vi "ELVIS III v1.0 Build Bitmask DIO.vi"(10 "bool Value List In":bool[](array[boolean]), 11 "Channel List":T3) -> (1 "Bitmask to Channel Array":T1[](array[typedef]), 2 "OUT Bitmask Array":bool[][](array[boolean]), 3 "DIR Bitmask Array":bool[][](array[boolean]))   [LabVIEW 2021]
uses:
  <vilib>/myRIO/Common/Instrument Driver Framework/myRIO v1.0/DIO/typedefs/DIO Channels List.ctl
  <vilib>/myRIO/Common/Instrument Driver Framework/myRIO v1.0/DIO/typedefs/DIO Channels Enum.ctl
  <vilib>/myRIO/Common/Instrument Driver Framework/ELVIS III v1.0/DIO/typedefs/ELVIS III DIO Bitmask to Channel Map.ctl
  <vilib>/myRIO/Common/Instrument Driver Framework/ELVIS III v1.0/DIO/typedefs/ELVIS III DIO Bank Enum.ctl
panel:
  # "This VI is used by both the myRIO v1.0 Read DIO and Write DIO VIs. \nIf a bool Value List in is provided the appropriate OUT Botmask Array will be generated, otherwise all values in the array will be false."
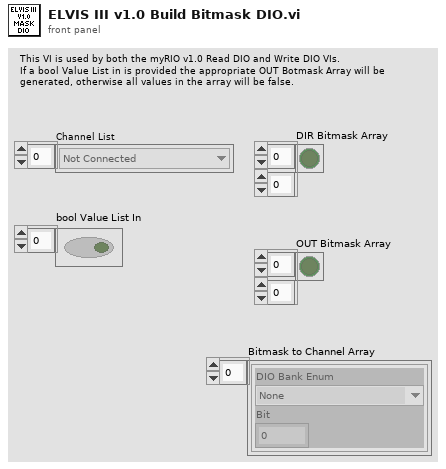
[diagram p1: front panel]
types:
  T1 = typedef "ELVIS III DIO Bitmask to Channel Map.ctl" = cluster{"DIO Bank Enum":T2, "Bit":i32}
  T2 = typedef "ELVIS III DIO Bank Enum.ctl" = enum32{"None", "A/DIO19:0", "B/DIO19:0", "LED3:0", "Button0"}
  T3 = typedef "DIO Channels List.ctl" = T4[]
  T4 = typedef "DIO Channels Enum.ctl" = enum16{"Not Connected", "C/DIO0", "C/DIO1", "C/DIO2", "C/DIO3", "C/DIO4", "C/DIO5", "C/DIO6", "C/DIO7", "A/DIO0", "A/DIO1", "A/DIO2", "A/DIO3", "A/DIO4", "A/DIO5", "A/DIO6", "A/DIO7", "A/DIO8", "A/DIO9", "A/DIO10", "A/DIO11", "A/DIO12", "A/DIO13", "A/DIO14", "A/DIO15", "A/DIO16", "A/DIO17", "A/DIO18", "A/DIO19", "B/DIO0", "B/DIO1", "B/DIO2", "B/DIO3", "B/DIO4", "B/DIO5", "B/DIO6", "B/DIO7", "B/DIO8", "B/DIO9", "B/DIO10", "B/DIO11", "B/DIO12", "B/DIO13", "B/DIO14", "B/DIO15", "B/DIO16", "B/DIO17", "B/DIO18", "B/DIO19", "LED0", "LED1", "LED2", "LED3", "Button0", "DIO/DIO0", "DIO/DIO1", "DIO/DIO2", "DIO/DIO3", "DIO/DIO4", "DIO/DIO5", "DIO/DIO6", "DIO/DIO7", "DIO/DIO8", "DIO/DIO9", "SPI/CS0", "SPI/CS1", "SPI/CS2", "SPI/CS3", "LED RADIO (Green)", "LED RADIO (Red)", "LED COMM (Green)", "LED COMM (Red)", "LED MODE (Green)", "LED MODE (Red)"}
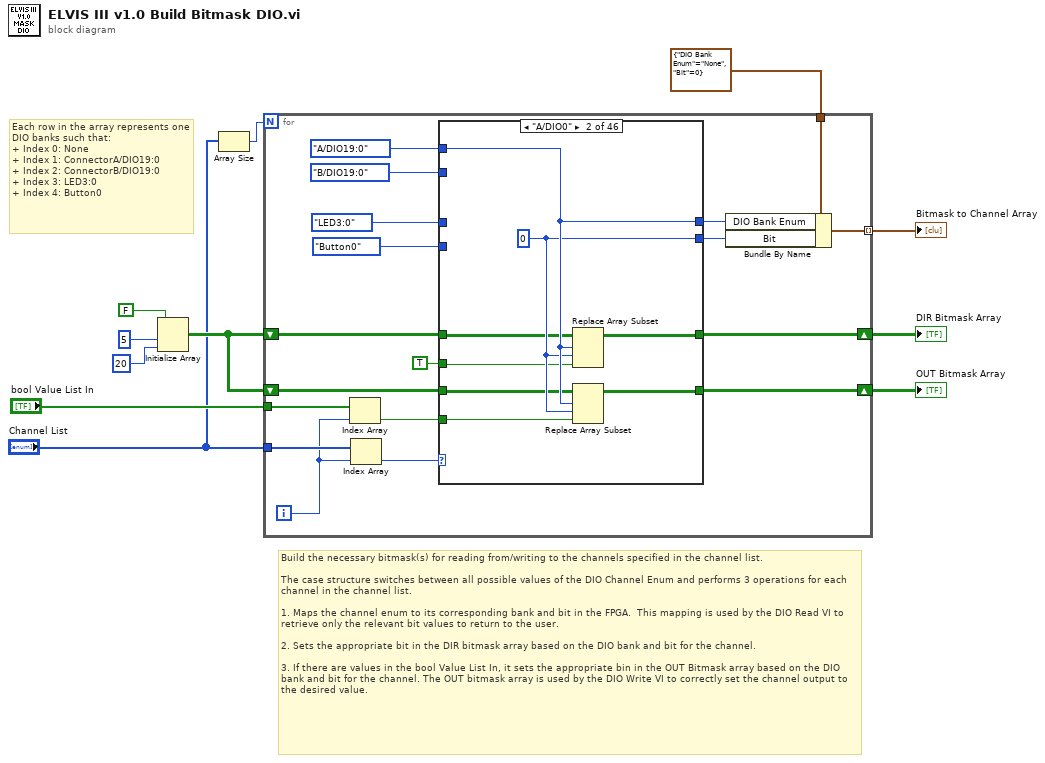
[diagram p0: block diagram]
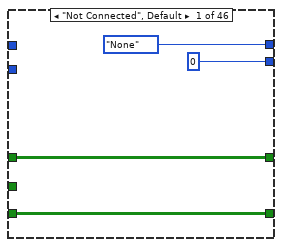
[diagram p2: hidden frame]
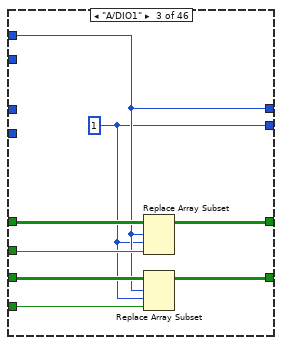
[diagram p3: hidden frame]
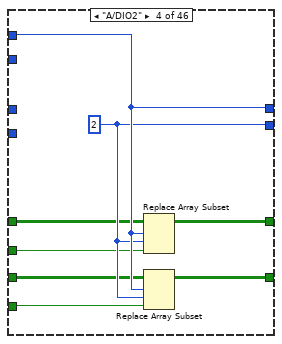
[diagram p4: hidden frame]
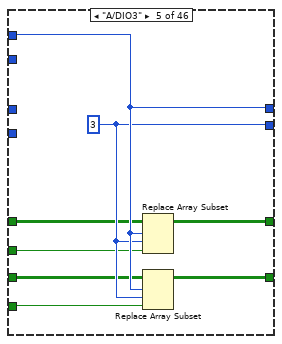
[diagram p5: hidden frame]
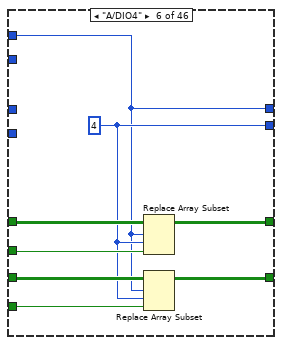
[diagram p6: hidden frame]
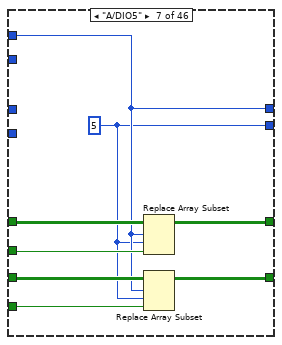
[diagram p7: hidden frame]
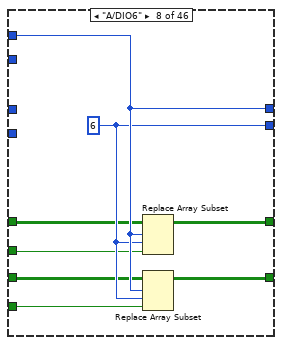
[diagram p8: hidden frame]
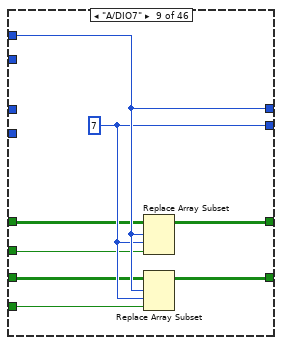
[diagram p9: hidden frame]
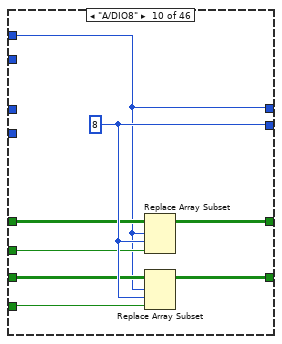
[diagram p10: hidden frame]
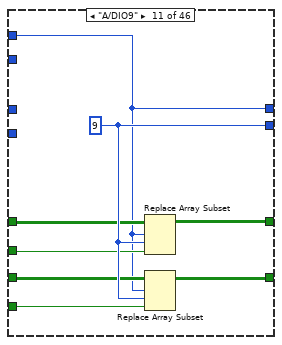
[diagram p11: hidden frame]
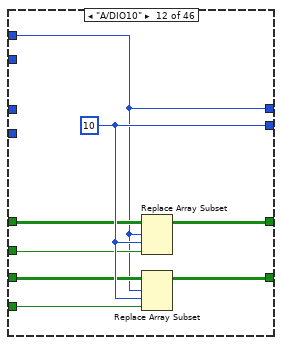
[diagram p12: hidden frame]
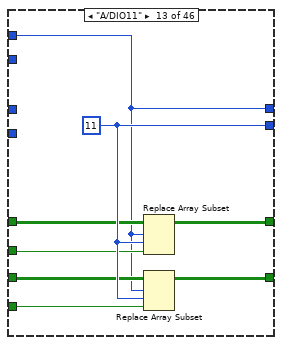
[diagram p13: hidden frame]
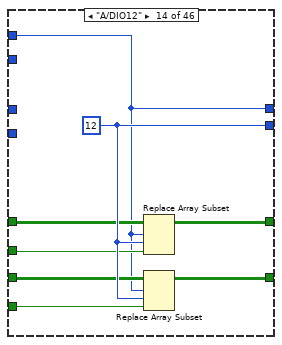
[diagram p14: hidden frame]
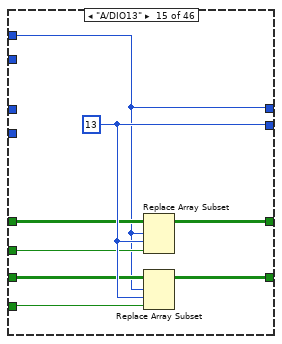
[diagram p15: hidden frame]
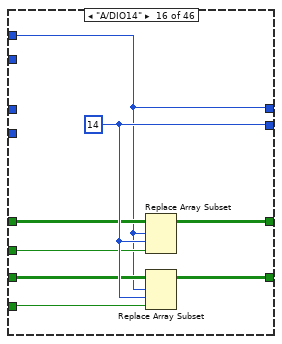
[diagram p16: hidden frame]
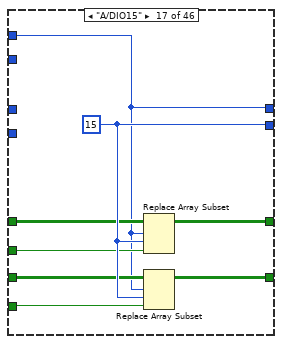
[diagram p17: hidden frame]
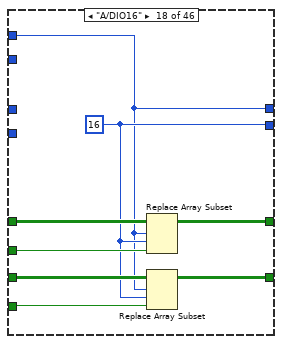
[diagram p18: hidden frame]
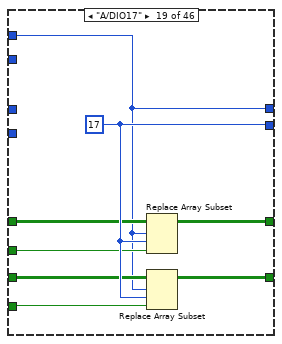
[diagram p19: hidden frame]
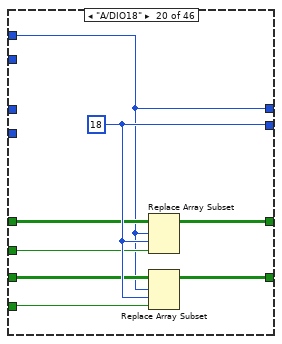
[diagram p20: hidden frame]
diagram:
  # "Build the necessary bitmask(s) for reading from/writing to the channels specified in the channel list.\n\nThe case structure switches between all possible values of the DIO Channel Enum and performs 3 operations for each channel in the channel list. \n\n1. Maps the channel enum to its corresponding bank and bit in the FPGA.  This mapping is used by the DIO Read VI to retrieve only the relevant bit values to return to the user.\n\n2. Sets the appropriate bit in the DIR bitmask array based on the DIO bank and bit for the channel.\n\n3. If there are values in the bool Value List In, it sets the appropriate bin in the OUT Bitmask array based on the DIO bank and bit for the channel. The OUT bitmask array is used by the DIO Write VI to correctly set the channel output to the desired value."
  # "Each row in the array represents one DIO banks such that:\n+ Index 0: None\n+ Index 1: ConnectorA/DIO19:0\n+ Index 2: ConnectorB/DIO19:0\n+ Index 3: LED3:0\n+ Index 4: Button0"
  n1 = Initialize Array(FALSE, 5 ("dimension size"), 20 ("dimension size")) -> (w6:bool[][])
  n2 = Array Size(array="Channel List") -> (size(s)=w3:i32)
  n3 = for {
    N: w3 -> [_]
    tunnel: "Channel List" -> [w20]
    shift-right: [w27] -> w10
    shift-left: w6 -> [w29]
    tunnel: T1 {"DIO Bank Enum"=enum."None", "Bit"=0} ("DIO Channel to Bitmask Map") -> [w15]
    tunnel: [w25] -> w7 mode=indexing
    shift-right: [w22] -> w5
    shift-left: w6 -> [w23]
    tunnel: "bool Value List In" -> [w21]
    i -> [w18]
    n4 = Index Array(array=w21, index=w18) -> (element=w17:bool)
    n5 = Index Array(array=w20, index=w18) -> (element=w19:T4)
    n6 = case shown="\"A/DIO0\"" w19 {
      tunnel: w29 -> [w33 w39 w49 w55 w63 w73 w81 w85 w93 w104 w112 w118 w126 w134 w144 w152 w160 w169 w174 w184 w190 w200 w206 w214 w222 w230 w238 w247 w256 w262 w270 w278 w288 w294 w302 w310 w318 w326 w334 w342 w350 w358 w365 w374 w381 w393]
      tunnel: TRUE ("new element/subarray") -> [_ w35 w48 w52 w62 w72 w80 w84 w92 w100 w111 w117 w125 w133 w140 w149 w159 w166 w173 w181 w189 w199 w205 w213 w221 w229 w237 w246 w255 w261 w269 w277 w287 w293 w301 w309 w317 w325 w333 w341 w349 w357 w364 w373 w380 w387]
      tunnel: [w33 w38 w46 w54 w59 w68 w75 w87 w95 w103 w107 w120 w128 w136 w143 w151 w155 w168 w176 w183 w192 w195 w208 w216 w224 w232 w240 w248 w254 w264 w272 w280 w283 w296 w304 w312 w320 w328 w336 w344 w352 w360 w367 w375 w383 w392] -> w27
      tunnel: [0 ("disabled index (col)") w40 w42 w56 w64 w67 w76 w88 w96 w105 w113 w121 w129 w137 w145 w153 w161 w163 w177 w185 w193 w201 w209 w217 w225 w233 w241 w249 w257 w265 w273 w281 w289 w297 w305 w313 w321 w329 w337 w345 w353 w361 w368 w376 w384 w389] -> w26
      tunnel: [ELVIS_III_DIO_Bank_Enum."None" ("DIO Bank Enum") w41 w43 w57 w65 w66 w77 w89 w97 w98 w106 w114 w122 w130 w138 w146 w154 w162 w170 w178 w186 w194 w202 w210 w218 w226 w234 w242 w250 w258 w266 w274 w282 w290 w298 w306 w314 w322 w330 w338 w346 w354 w369 w377 w385 w388] -> w24
      tunnel: w23 -> [w31 w36 w45 w51 w61 w71 w79 w83 w91 w101 w110 w116 w124 w132 w141 w148 w158 w165 w172 w180 w188 w198 w204 w212 w220 w228 w236 w245 w252 w260 w268 w276 w286 w292 w300 w308 w316 w324 w332 w340 w348 w356 w363 w372 w379 w391]
      tunnel: [w31 w37 w47 w53 w58 w69 w74 w86 w94 w102 w108 w119 w127 w135 w142 w150 w156 w167 w175 w182 w191 w196 w207 w215 w223 w231 w239 w243 w253 w263 w271 w279 w284 w295 w303 w311 w319 w327 w335 w343 w351 w359 w366 w371 w382 w390] -> w22
      tunnel: w17 -> [_ w34 w44 w50 w60 w70 w78 w82 w90 w99 w109 w115 w123 w131 w139 w147 w157 w164 w171 w179 w187 w197 w203 w211 w219 w227 w235 w244 w251 w259 w267 w275 w285 w291 w299 w307 w315 w323 w331 w339 w347 w355 w362 w370 w378 w386]
      tunnel: ELVIS_III_DIO_Bank_Enum."A/DIO19:0" ("DIO Bank Enum") -> [_ w41 w43 w57 w65 w66 w77 w89 w97 w98 w106 w114 w122 w130 w138 w146 w154 w162 w170 w178 w186 _ _ _ _ _ _ _ _ _ _ _ _ _ _ _ _ _ _ _ _ _ _ _ _ _]
      tunnel: ELVIS_III_DIO_Bank_Enum."B/DIO19:0" ("DIO Bank Enum") -> [_ _ _ _ _ _ _ _ _ _ _ _ _ _ _ _ _ _ _ _ _ w194 w202 w210 w218 w226 w234 w242 w250 w258 w266 w274 w282 w290 w298 w306 w314 w322 w330 w338 w346 _ _ _ _ _]
      tunnel: ELVIS_III_DIO_Bank_Enum."Button0" ("DIO Bank Enum") -> [_ _ _ _ _ _ _ _ _ _ _ _ _ _ _ _ _ _ _ _ _ _ _ _ _ _ _ _ _ _ _ _ _ _ _ _ _ _ _ _ _ _ _ _ _ w388]
      tunnel: ELVIS_III_DIO_Bank_Enum."LED3:0" ("DIO Bank Enum") -> [_ _ _ _ _ _ _ _ _ _ _ _ _ _ _ _ _ _ _ _ _ _ _ _ _ _ _ _ _ _ _ _ _ _ _ _ _ _ _ _ _ w354 w369 w377 w385 _]
      frame "Not Connected", Default {
      }
      frame "A/DIO0" {
        w40 = 0 ("disabled index (col)")
        n7 = Replace Array Subset(array=w39, new element=w35, index (row)=w41, index (col)=w40) -> (w38:bool[][])
        n8 = Replace Array Subset(array=w36, new element=w34, index (row)=w41, index (col)=w40) -> (w37:bool[][])
      }
      frame "A/DIO1" {
        w42 = 1 ("disabled index (col)")
        n9 = Replace Array Subset(array=w49, new element=w48, index (row)=w43, index (col)=w42) -> (w46:bool[][])
        n10 = Replace Array Subset(array=w45, new element=w44, index (row)=w43, index (col)=w42) -> (w47:bool[][])
      }
      frame "A/DIO2" {
        w56 = 2 ("disabled index (col)")
        n11 = Replace Array Subset(array=w55, new element=w52, index (row)=w57, index (col)=w56) -> (w54:bool[][])
        n12 = Replace Array Subset(array=w51, new element=w50, index (row)=w57, index (col)=w56) -> (w53:bool[][])
      }
      frame "A/DIO3" {
        w64 = 3 ("disabled index (col)")
        n13 = Replace Array Subset(array=w63, new element=w62, index (row)=w65, index (col)=w64) -> (w59:bool[][])
        n14 = Replace Array Subset(array=w61, new element=w60, index (row)=w65, index (col)=w64) -> (w58:bool[][])
      }
      frame "A/DIO4" {
        w67 = 4 ("disabled index (col)")
        n15 = Replace Array Subset(array=w73, new element=w72, index (row)=w66, index (col)=w67) -> (w68:bool[][])
        n16 = Replace Array Subset(array=w71, new element=w70, index (row)=w66, index (col)=w67) -> (w69:bool[][])
      }
      frame "A/DIO5" {
        w76 = 5 ("disabled index (col)")
        n17 = Replace Array Subset(array=w81, new element=w80, index (row)=w77, index (col)=w76) -> (w75:bool[][])
        n18 = Replace Array Subset(array=w79, new element=w78, index (row)=w77, index (col)=w76) -> (w74:bool[][])
      }
      frame "A/DIO6" {
        w88 = 6 ("disabled index (col)")
        n19 = Replace Array Subset(array=w85, new element=w84, index (row)=w89, index (col)=w88) -> (w87:bool[][])
        n20 = Replace Array Subset(array=w83, new element=w82, index (row)=w89, index (col)=w88) -> (w86:bool[][])
      }
      frame "A/DIO7" {
        w96 = 7 ("disabled index (col)")
        n21 = Replace Array Subset(array=w93, new element=w92, index (row)=w97, index (col)=w96) -> (w95:bool[][])
        n22 = Replace Array Subset(array=w91, new element=w90, index (row)=w97, index (col)=w96) -> (w94:bool[][])
      }
      frame "A/DIO8" {
        w105 = 8 ("disabled index (col)")
        n23 = Replace Array Subset(array=w104, new element=w100, index (row)=w98, index (col)=w105) -> (w103:bool[][])
        n24 = Replace Array Subset(array=w101, new element=w99, index (row)=w98, index (col)=w105) -> (w102:bool[][])
      }
      frame "A/DIO9" {
        w113 = 9 ("disabled index (col)")
        n25 = Replace Array Subset(array=w112, new element=w111, index (row)=w106, index (col)=w113) -> (w107:bool[][])
        n26 = Replace Array Subset(array=w110, new element=w109, index (row)=w106, index (col)=w113) -> (w108:bool[][])
      }
      frame "A/DIO10" {
        w121 = 10 ("disabled index (col)")
        n27 = Replace Array Subset(array=w118, new element=w117, index (row)=w114, index (col)=w121) -> (w120:bool[][])
        n28 = Replace Array Subset(array=w116, new element=w115, index (row)=w114, index (col)=w121) -> (w119:bool[][])
      }
      frame "A/DIO11" {
        w129 = 11 ("disabled index (col)")
        n29 = Replace Array Subset(array=w126, new element=w125, index (row)=w122, index (col)=w129) -> (w128:bool[][])
        n30 = Replace Array Subset(array=w124, new element=w123, index (row)=w122, index (col)=w129) -> (w127:bool[][])
      }
      frame "A/DIO12" {
        w137 = 12 ("disabled index (col)")
        n31 = Replace Array Subset(array=w134, new element=w133, index (row)=w130, index (col)=w137) -> (w136:bool[][])
        n32 = Replace Array Subset(array=w132, new element=w131, index (row)=w130, index (col)=w137) -> (w135:bool[][])
      }
      frame "A/DIO13" {
        w145 = 13 ("disabled index (col)")
        n33 = Replace Array Subset(array=w144, new element=w140, index (row)=w138, index (col)=w145) -> (w143:bool[][])
        n34 = Replace Array Subset(array=w141, new element=w139, index (row)=w138, index (col)=w145) -> (w142:bool[][])
      }
      frame "A/DIO14" {
        w153 = 14 ("disabled index (col)")
        n35 = Replace Array Subset(array=w152, new element=w149, index (row)=w146, index (col)=w153) -> (w151:bool[][])
        n36 = Replace Array Subset(array=w148, new element=w147, index (row)=w146, index (col)=w153) -> (w150:bool[][])
      }
      frame "A/DIO15" {
        w161 = 15 ("disabled index (col)")
        n37 = Replace Array Subset(array=w160, new element=w159, index (row)=w154, index (col)=w161) -> (w155:bool[][])
        n38 = Replace Array Subset(array=w158, new element=w157, index (row)=w154, index (col)=w161) -> (w156:bool[][])
      }
      frame "A/DIO16" {
        w163 = 16 ("disabled index (col)")
        n39 = Replace Array Subset(array=w169, new element=w166, index (row)=w162, index (col)=w163) -> (w168:bool[][])
        n40 = Replace Array Subset(array=w165, new element=w164, index (row)=w162, index (col)=w163) -> (w167:bool[][])
      }
      frame "A/DIO17" {
        w177 = 17 ("disabled index (col)")
        n41 = Replace Array Subset(array=w174, new element=w173, index (row)=w170, index (col)=w177) -> (w176:bool[][])
        n42 = Replace Array Subset(array=w172, new element=w171, index (row)=w170, index (col)=w177) -> (w175:bool[][])
      }
      frame "A/DIO18" {
        w185 = 18 ("disabled index (col)")
        n43 = Replace Array Subset(array=w184, new element=w181, index (row)=w178, index (col)=w185) -> (w183:bool[][])
        n44 = Replace Array Subset(array=w180, new element=w179, index (row)=w178, index (col)=w185) -> (w182:bool[][])
      }
      frame "A/DIO19" {
        w193 = 19 ("disabled index (col)")
        n45 = Replace Array Subset(array=w190, new element=w189, index (row)=w186, index (col)=w193) -> (w192:bool[][])
        n46 = Replace Array Subset(array=w188, new element=w187, index (row)=w186, index (col)=w193) -> (w191:bool[][])
      }
      frame "B/DIO0" {
        w201 = 0 ("disabled index (col)")
        n47 = Replace Array Subset(array=w200, new element=w199, index (row)=w194, index (col)=w201) -> (w195:bool[][])
        n48 = Replace Array Subset(array=w198, new element=w197, index (row)=w194, index (col)=w201) -> (w196:bool[][])
      }
      frame "B/DIO1" {
        w209 = 1 ("disabled index (col)")
        n49 = Replace Array Subset(array=w206, new element=w205, index (row)=w202, index (col)=w209) -> (w208:bool[][])
        n50 = Replace Array Subset(array=w204, new element=w203, index (row)=w202, index (col)=w209) -> (w207:bool[][])
      }
      frame "B/DIO2" {
        w217 = 2 ("disabled index (col)")
        n51 = Replace Array Subset(array=w214, new element=w213, index (row)=w210, index (col)=w217) -> (w216:bool[][])
        n52 = Replace Array Subset(array=w212, new element=w211, index (row)=w210, index (col)=w217) -> (w215:bool[][])
      }
      frame "B/DIO3" {
        w225 = 3 ("disabled index (col)")
        n53 = Replace Array Subset(array=w222, new element=w221, index (row)=w218, index (col)=w225) -> (w224:bool[][])
        n54 = Replace Array Subset(array=w220, new element=w219, index (row)=w218, index (col)=w225) -> (w223:bool[][])
      }
      frame "B/DIO4" {
        w233 = 4 ("disabled index (col)")
        n55 = Replace Array Subset(array=w230, new element=w229, index (row)=w226, index (col)=w233) -> (w232:bool[][])
        n56 = Replace Array Subset(array=w228, new element=w227, index (row)=w226, index (col)=w233) -> (w231:bool[][])
      }
      frame "B/DIO5" {
        w241 = 5 ("disabled index (col)")
        n57 = Replace Array Subset(array=w238, new element=w237, index (row)=w234, index (col)=w241) -> (w240:bool[][])
        n58 = Replace Array Subset(array=w236, new element=w235, index (row)=w234, index (col)=w241) -> (w239:bool[][])
      }
      frame "B/DIO6" {
        w249 = 6 ("disabled index (col)")
        n59 = Replace Array Subset(array=w247, new element=w246, index (row)=w242, index (col)=w249) -> (w248:bool[][])
        n60 = Replace Array Subset(array=w245, new element=w244, index (row)=w242, index (col)=w249) -> (w243:bool[][])
      }
      frame "B/DIO7" {
        w257 = 7 ("disabled index (col)")
        n61 = Replace Array Subset(array=w256, new element=w255, index (row)=w250, index (col)=w257) -> (w254:bool[][])
        n62 = Replace Array Subset(array=w252, new element=w251, index (row)=w250, index (col)=w257) -> (w253:bool[][])
      }
      frame "B/DIO8" {
        w265 = 8 ("disabled index (col)")
        n63 = Replace Array Subset(array=w262, new element=w261, index (row)=w258, index (col)=w265) -> (w264:bool[][])
        n64 = Replace Array Subset(array=w260, new element=w259, index (row)=w258, index (col)=w265) -> (w263:bool[][])
      }
      frame "B/DIO9" {
        w273 = 9 ("disabled index (col)")
        n65 = Replace Array Subset(array=w270, new element=w269, index (row)=w266, index (col)=w273) -> (w272:bool[][])
        n66 = Replace Array Subset(array=w268, new element=w267, index (row)=w266, index (col)=w273) -> (w271:bool[][])
      }
      frame "B/DIO10" {
        w281 = 10 ("disabled index (col)")
        n67 = Replace Array Subset(array=w278, new element=w277, index (row)=w274, index (col)=w281) -> (w280:bool[][])
        n68 = Replace Array Subset(array=w276, new element=w275, index (row)=w274, index (col)=w281) -> (w279:bool[][])
      }
      frame "B/DIO11" {
        w289 = 11 ("disabled index (col)")
        n69 = Replace Array Subset(array=w288, new element=w287, index (row)=w282, index (col)=w289) -> (w283:bool[][])
        n70 = Replace Array Subset(array=w286, new element=w285, index (row)=w282, index (col)=w289) -> (w284:bool[][])
      }
      frame "B/DIO12" {
        w297 = 12 ("disabled index (col)")
        n71 = Replace Array Subset(array=w294, new element=w293, index (row)=w290, index (col)=w297) -> (w296:bool[][])
        n72 = Replace Array Subset(array=w292, new element=w291, index (row)=w290, index (col)=w297) -> (w295:bool[][])
      }
      frame "B/DIO13" {
        w305 = 13 ("disabled index (col)")
        n73 = Replace Array Subset(array=w302, new element=w301, index (row)=w298, index (col)=w305) -> (w304:bool[][])
        n74 = Replace Array Subset(array=w300, new element=w299, index (row)=w298, index (col)=w305) -> (w303:bool[][])
      }
      frame "B/DIO14" {
        w313 = 14 ("disabled index (col)")
        n75 = Replace Array Subset(array=w310, new element=w309, index (row)=w306, index (col)=w313) -> (w312:bool[][])
        n76 = Replace Array Subset(array=w308, new element=w307, index (row)=w306, index (col)=w313) -> (w311:bool[][])
      }
      frame "B/DIO15" {
        w321 = 15 ("disabled index (col)")
        n77 = Replace Array Subset(array=w318, new element=w317, index (row)=w314, index (col)=w321) -> (w320:bool[][])
        n78 = Replace Array Subset(array=w316, new element=w315, index (row)=w314, index (col)=w321) -> (w319:bool[][])
      }
      frame "B/DIO16" {
        w329 = 16 ("disabled index (col)")
        n79 = Replace Array Subset(array=w326, new element=w325, index (row)=w322, index (col)=w329) -> (w328:bool[][])
        n80 = Replace Array Subset(array=w324, new element=w323, index (row)=w322, index (col)=w329) -> (w327:bool[][])
      }
      frame "B/DIO17" {
        w337 = 17 ("disabled index (col)")
        n81 = Replace Array Subset(array=w334, new element=w333, index (row)=w330, index (col)=w337) -> (w336:bool[][])
        n82 = Replace Array Subset(array=w332, new element=w331, index (row)=w330, index (col)=w337) -> (w335:bool[][])
      }
      frame "B/DIO18" {
        w345 = 18 ("disabled index (col)")
        n83 = Replace Array Subset(array=w342, new element=w341, index (row)=w338, index (col)=w345) -> (w344:bool[][])
        n84 = Replace Array Subset(array=w340, new element=w339, index (row)=w338, index (col)=w345) -> (w343:bool[][])
      }
      frame "B/DIO19" {
        w353 = 19 ("disabled index (col)")
        n85 = Replace Array Subset(array=w350, new element=w349, index (row)=w346, index (col)=w353) -> (w352:bool[][])
        n86 = Replace Array Subset(array=w348, new element=w347, index (row)=w346, index (col)=w353) -> (w351:bool[][])
      }
      frame "LED0" {
        w361 = 0 ("disabled index (col)")
        n87 = Replace Array Subset(array=w358, new element=w357, index (row)=w354, index (col)=w361) -> (w360:bool[][])
        n88 = Replace Array Subset(array=w356, new element=w355, index (row)=w354, index (col)=w361) -> (w359:bool[][])
      }
      frame "LED1" {
        w368 = 1 ("disabled index (col)")
        n89 = Replace Array Subset(array=w365, new element=w364, index (row)=w369, index (col)=w368) -> (w367:bool[][])
        n90 = Replace Array Subset(array=w363, new element=w362, index (row)=w369, index (col)=w368) -> (w366:bool[][])
      }
      frame "LED2" {
        w376 = 2 ("disabled index (col)")
        n91 = Replace Array Subset(array=w374, new element=w373, index (row)=w377, index (col)=w376) -> (w375:bool[][])
        n92 = Replace Array Subset(array=w372, new element=w370, index (row)=w377, index (col)=w376) -> (w371:bool[][])
      }
      frame "LED3" {
        w384 = 3 ("disabled index (col)")
        n93 = Replace Array Subset(array=w381, new element=w380, index (row)=w385, index (col)=w384) -> (w383:bool[][])
        n94 = Replace Array Subset(array=w379, new element=w378, index (row)=w385, index (col)=w384) -> (w382:bool[][])
      }
      frame "Button0" {
        w389 = 0 ("disabled index (col)")
        n95 = Replace Array Subset(array=w393, new element=w387, index (row)=w388, index (col)=w389) -> (w392:bool[][])
        n96 = Replace Array Subset(array=w391, new element=w386, index (row)=w388, index (col)=w389) -> (w390:bool[][])
      }
    }
    n97 = Bundle By Name(cluster=w15, "DIO Bank Enum"=w24, "Bit"=w26) -> (w25:T1)
  }
  "DIR Bitmask Array" <- w10
  "Bitmask to Channel Array" <- w7
  "OUT Bitmask Array" <- w5
